vi "全局-配置识别.vi"() -> ()   [LabVIEW 2019]
panel:
  in  "主发等待":u32
  in  "停止":bool
  in  "等待延迟":u32
  in  "空强制延时":u32
  out "连接":string
  out "模式":string
  # "全局变量\n用于在通讯中判断当前连接"
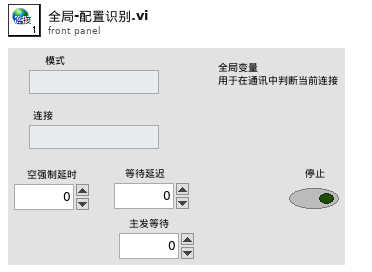
[diagram p1: front panel]
diagram:
